vi "Update Steering to Wheel Frame Transform.vi"(5 "x wheel position":dbl, 7 "y wheel position":dbl, 8 "error in (no error)":errorcluster, 9 "wheel frame angle (rad)":dbl, 11 "wheel in":refnum<class "NI_Robotics_Wheel.lvclass">) -> (0 "error out":errorcluster, 3 "wheel out":refnum<class "NI_Robotics_Wheel.lvclass">)   [LabVIEW 2017, in "NI_Robotics_Wheel.lvclass"]
uses:
  <vilib>/robotics/Steering/Wheel/NI_Robotics_Wheel.lvclass
  <vilib>/robotics/Steering/Wheel/NI_Robotics_Wheel.lvclass/NI_Robotics_Wheel.ctl
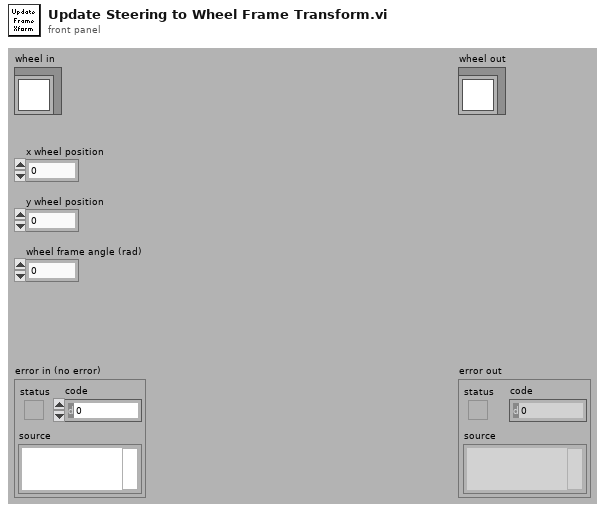
[diagram p1: front panel]
types:
  T1 = typedef "NI_Matrix.lvlib/RealMatrix.ctl" = dbl[][]
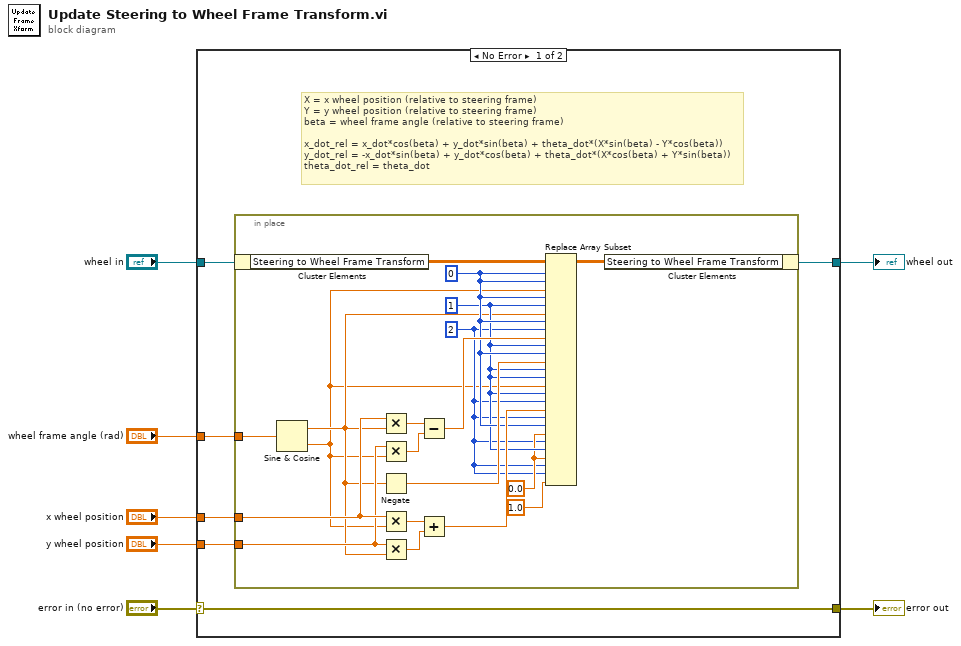
[diagram p0: block diagram]
diagram:
  n1 = case shown="No Error" "error in (no error)" {
    selector: "error in (no error)" -> [w13 w34]
    tunnel: [w13 w34] -> w6
    tunnel: [w11 w33] -> w4
    tunnel: "wheel in" -> [w12 w33]
    tunnel: "wheel frame angle (rad)" -> [w10 _]
    tunnel: "x wheel position" -> [w9 _]
    tunnel: "y wheel position" -> [w8 _]
    frame No Error {
      # "X = x wheel position (relative to steering frame)\nY = y wheel position (relative to steering frame)\nbeta = wheel frame angle (relative to steering frame)\n\nx_dot_rel = x_dot*cos(beta) + y_dot*sin(beta) + theta_dot*(X*sin(beta) - Y*cos(beta))\ny_dot_rel = -x_dot*sin(beta) + y_dot*cos(beta) + theta_dot*(X*cos(beta) + Y*sin(beta))\ntheta_dot_rel = theta_dot"
      n2 = in-place {
        in-place-border: w10 -> [w16]
        in-place-border: w9 -> [w23]
        in-place-border: w8 -> [w22]
        w19 = 0.0 ("new element/subarray")
        w18 = 2 ("disabled index (col)")
        w20 = 1 ("disabled index (col)")
        w21 = 0 ("index (row)")
        n3 = in-place-cluster #1(w12) -> ("Steering to Wheel Frame Transform"=w25:T1)
        n4 = Sine & Cosine(0:w16) -> (1:w15:dbl, 2:w14:dbl)
        n5 = Multiply(x=w23, y=w15) -> (x*y=w29:dbl)
        n6 = Multiply(x=w22, y=w14) -> (x*y=w28:dbl)
        n7 = Negate(x=w15) -> (-x=w31:dbl)
        n8 = Multiply(x=w23, y=w14) -> (x*y=w27:dbl)
        n9 = Multiply(x=w22, y=w15) -> (x*y=w26:dbl)
        n10 = Subtract(x=w29, y=w28) -> (x-y=w30:dbl)
        n11 = Add(x=w27, y=w26) -> (x+y=w32:dbl)
        n12 = Replace Array Subset(array=w25, new element #1=w14, index (row) #1=w21, index (col) #1=w21, new element #2=w15, index (row) #2=w21, index (col) #2=w20, new element #3=w30, index (row) #3=w21, index (col) #3=w18, new element #4=w31, index (row) #4=w20, index (col) #4=w21, new element #5=w14, index (row) #5=w20, index (col) #5=w20, new element #6=w32, index (row) #6=w20, index (col) #6=w18, new element #7=w19, index (row) #7=w18, index (col) #7=w21, new element #8=w19, index (row) #8=w18, index (col) #8=w20, new element #9=1.0 ("new element/subarray"), index (row) #9=w18, index (col) #9=w18) -> (w24:T1)
        n13 = in-place-cluster #1("Steering to Wheel Frame Transform"=w24) -> (w11:refnum<class "NI_Robotics_Wheel.lvclass">)
      }
    }
    frame Error {
    }
  }
  "error out" <- w6
  "wheel out" <- w4
